vi "sensor cmd state status.vi"(9 "dest":u16, 10 "v2_state_id":u32, 11 "device_handle":u32) -> (1 "dest out":u16, 2 "function return":i32, 3 "device_handle out":u32)   [LabVIEW 2019, in "apdm.lvlib"]
doc: "APDM_EXPORT int apdm_sensor_cmd_state_status(apdm_device_handle_t device_handle, const uint32_t v2_state_id, uint16_t *dest);"
uses:
  apdm.lvlib
  Lee Lab/CP FES Walking 2018/Code/Working/LabVIEW/apdm.dll
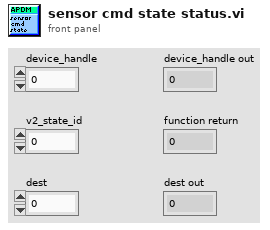
[diagram p1: front panel]
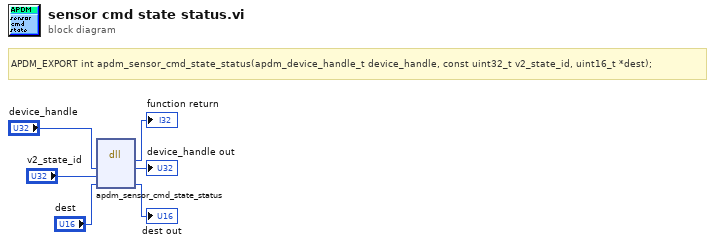
[diagram p0: block diagram]
diagram:
  # "APDM_EXPORT int apdm_sensor_cmd_state_status(apdm_device_handle_t device_handle, const uint32_t v2_state_id, uint16_t *dest);"
  n1 = dll-call lib="C:/Users/jfalesi/Dropbox/Lee Lab/CP FES Walking 2018/Code/Working/LabVIEW/apdm.*" fn="apdm_sensor_cmd_state_status"("device_handle"="device_handle", "v2_state_id"="v2_state_id", "dest"="dest") -> (→"function return":i32, "device_handle"=→"device_handle out":u32, "dest"=→"dest out":u16)  [unwired: 4 in, 2 out]
